vi "Enque(RunTest).vi"(7 "at front (F)":bool, 8 "error in":errorcluster, 9 "RunTest":T1, 10 "Message Command":string="StartTestSequence", 11 "Message que":T2) -> (0 "error out":errorcluster, 3 "Message que out":T2)   [LabVIEW 2019]
doc: "Transmit a message with a string payload.\nFor a regular message, enqueue the message. For a priority message, enqueue it at the front of the queue.\n\nBolder Software LLC"
uses:
  MessageQue/MessageQue.ctl
  MessageQue/MessageCluster.ctl
  RunTest.ctl
  MessageQue/MessageQue.lvlib
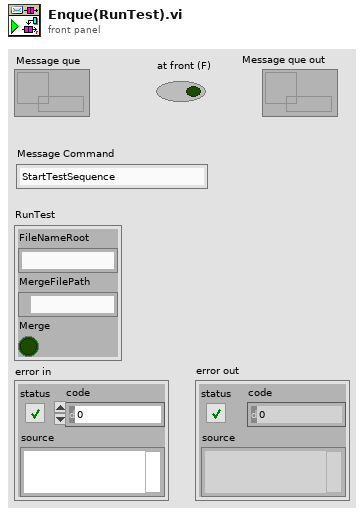
[diagram p1: front panel]
types:
  T1 = typedef "RunTest.ctl" = cluster{"FileNameRoot":string, "MergeFilePath":path, "Merge":bool}
  T2 = typedef "MessageQue.lvlib/MessageQue.ctl" = refnum<queue>
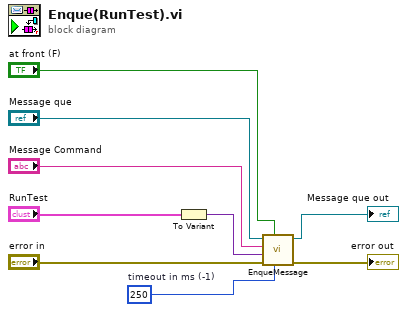
[diagram p0: block diagram]
diagram:
  w9 = 250  # timeout in ms (-1)
  n1 = To Variant(anything="RunTest") -> (Variant=w3:variant)
  n2 = call "EnqueMessage.vi"("timeout in ms (-1)"=w9, "Priority Message? (F)"="at front (F)", "error in"="error in", "Message Payload"=w3, "Message Command"="Message Command", "Message que"="Message que") -> ("error out"=→"error out":errorcluster, "Message que out"=→"Message que out":T2)  [unwired: 4 in]
